vi "running linear fit.vi"() -> ()   [LabVIEW 2019]
uses:
  <vilib>/ptbypt/NI_PtbyPt.lvlib
  <vilib>/Analysis/NI_AALBase.lvlib
panel:
  out "Array":dbl[](array[numeric])
  out "slope":dynamicdata(graph)
  out "Waveform Chart":dbl[](graph)
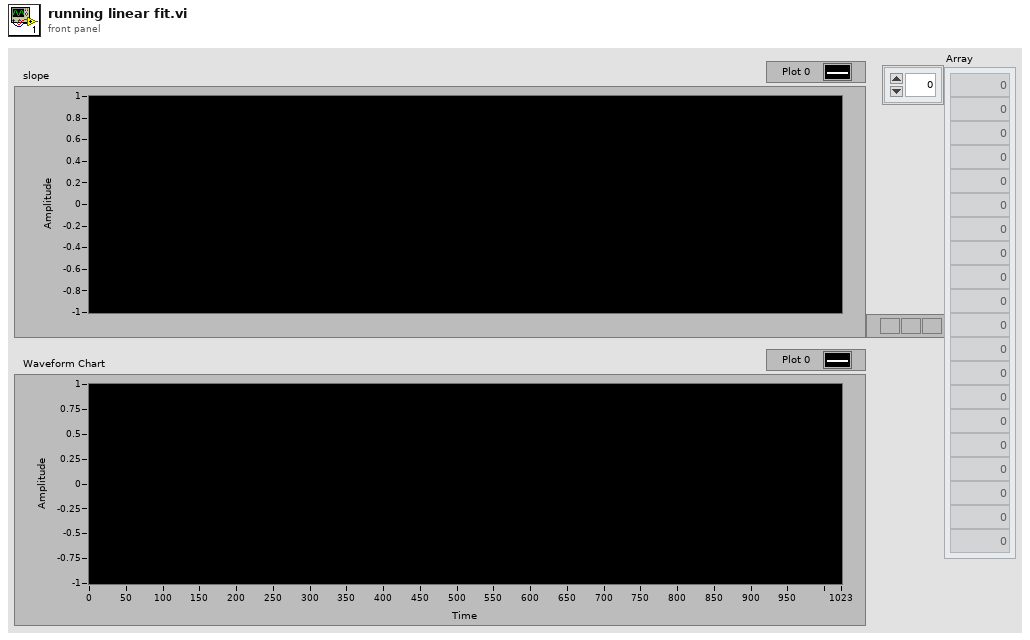
[diagram p1: front panel]
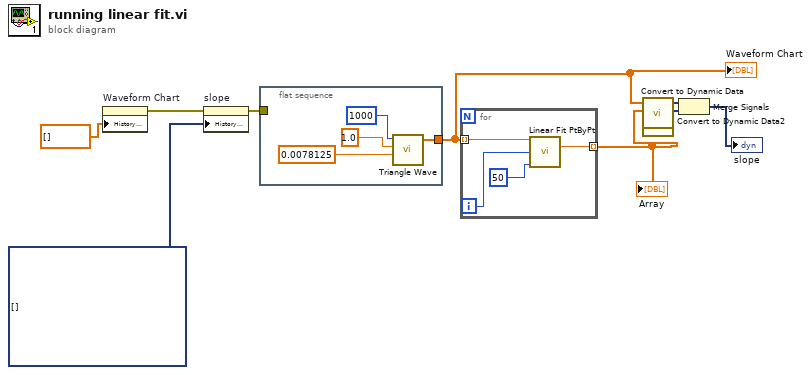
[diagram p0: block diagram]
diagram:
  n1 = property on="Waveform Chart" class="WFChart (strict)"("History Data"=dbl[] []) -> (error out=w9:errorcluster)  [unwired: 2 in, 1 out]
  n2 = property on="slope" class="WFChart (strict)"(error in=w9, "History Data"=dynamicdata[] []) -> (error out=w7:errorcluster)  [unwired: 1 in, 1 out]
  n3 = flat-sequence {
    tunnel: [w10] -> w6
    tunnel: w7 -> [_]
    frame #0 {
      n4 = call <vilib>:"Triangle Wave.vi"("samples"=1000, "amplitude"=1.0, "frequency"=0.0078125) -> ("triangle wave"=w10:dbl[])  [unwired: 2 in, 2 out]
    }
  }
  n5 = for {
    tunnel: w6 -> [w16] mode=indexing
    tunnel: [w15] -> w4 mode=indexing
    i -> [w14]
    n6 = call <vilib>:"Linear Fit PtByPt.vi"("y"=w16, "x"=w14, "sample length"=50) -> ("slope"=w15:dbl)  [unwired: 8 in, 4 out]
  }
  "Array" <- w4
  n7 = call "Convert to Dynamic Data"("Array"=w6) -> ("Dynamic Data Type"=w5:dynamicdata)  [unwired: 3 in]
  n8 = call "Convert to Dynamic Data2"("Array"=w4) -> ("Dynamic Data Type"=w3:dynamicdata)  [unwired: 3 in]
  n9 = Merge Signals(w5, w3) -> (→"slope":dynamicdata)
  "Waveform Chart" <- w6
